vi "UpdatingCount_RC.vi"(8 "error in":errorcluster, 10 "CountDetails":T1, 11 "Pass/Fail":bool) -> (0 "error out":errorcluster, 1 "Reel Counter Result":T2, 2 "Total Cluster Result":T3, 3 "CountDetailsOut":T1)   [LabVIEW 2019, in "Rack Controller.lvclass"]
uses:
  Rack Controller.lvclass
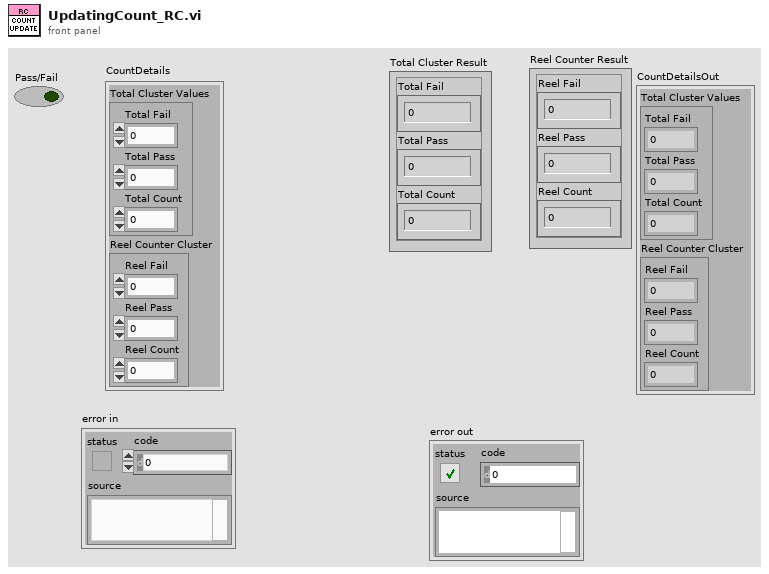
[diagram p1: front panel]
types:
  T1 = cluster{"Total Cluster Values":cluster{"Total Fail":u64, "Total Pass":u64, "Total Count":u64}, "Reel Counter Cluster":cluster{"Reel Fail":u64, "Reel Pass":u64, "Reel Count":u64}}
  T2 = cluster{"Reel Fail":u64, "Reel Pass":u64, "Reel Count":u64}
  T3 = cluster{"Total Fail":u64, "Total Pass":u64, "Total Count":u64}
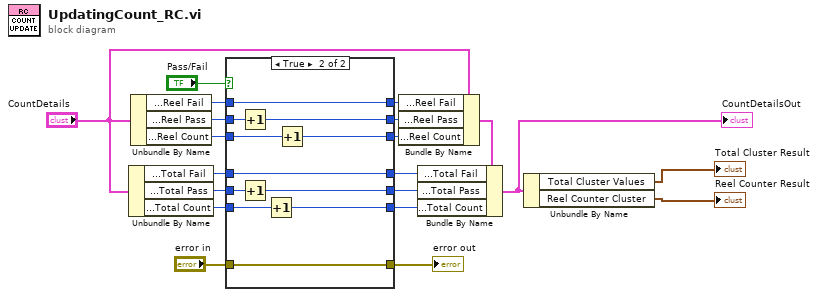
[diagram p0: block diagram]
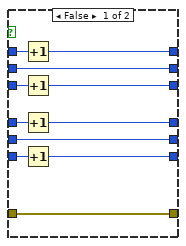
[diagram p2: hidden frame]
diagram:
  n1 = Unbundle By Name("CountDetails") -> ("Total Cluster Values.Total Fail"=w16:u64, "Total Cluster Values.Total Pass"=w17:u64, "Total Cluster Values.Total Count"=w18:u64)
  n2 = Unbundle By Name("CountDetails") -> ("Reel Counter Cluster.Reel Fail"=w12:u64, "Reel Counter Cluster.Reel Pass"=w11:u64, "Reel Counter Cluster.Reel Count"=w10:u64)
  n3 = case shown="True" "Pass/Fail" {
    tunnel: w17 -> [w31 w42]
    tunnel: w18 -> [w30 w41]
    tunnel: [w31 w40] -> w19
    tunnel: [w29 w32] -> w20
    tunnel: w16 -> [w28 w33]
    tunnel: [w27 w33] -> w15
    tunnel: [w26 w39] -> w14
    tunnel: "error in" -> [w26 w39]
    tunnel: w12 -> [w23 w35]
    tunnel: w11 -> [w21 w38]
    tunnel: w10 -> [w25 w36]
    tunnel: [w22 w35] -> w9
    tunnel: [w21 w37] -> w8
    tunnel: [w24 w34] -> w7
    frame False {
      n4 = Increment(x=w23) -> (x+1=w22:u64)
      n5 = Increment(x=w25) -> (x+1=w24:u64)
      n6 = Increment(x=w28) -> (x+1=w27:u64)
      n7 = Increment(x=w30) -> (x+1=w29:u64)
    }
    frame True {
      n8 = Increment(x=w38) -> (x+1=w37:u64)
      n9 = Increment(x=w42) -> (x+1=w40:u64)
      n10 = Increment(x=w41) -> (x+1=w32:u64)
      n11 = Increment(x=w36) -> (x+1=w34:u64)
    }
  }
  "error out" <- w14
  n12 = Bundle By Name(cluster="CountDetails", "Reel Counter Cluster.Reel Fail"=w9, "Reel Counter Cluster.Reel Pass"=w8, "Reel Counter Cluster.Reel Count"=w7) -> (w3:T1)
  n13 = Bundle By Name(cluster=w3, "Total Cluster Values.Total Fail"=w15, "Total Cluster Values.Total Pass"=w19, "Total Cluster Values.Total Count"=w20) -> (w2:T1)
  "CountDetailsOut" <- w2
  n14 = Unbundle By Name(w2) -> ("Total Cluster Values"=→"Total Cluster Result":T3, "Reel Counter Cluster"=→"Reel Counter Result":T2)
